vi "T3AWG Setup.vi"(4 "exact setup (True)":bool=TRUE, 5 "fs [Hz]":dbl=1000000000.0, 6 "N":i32, 7 "f [Hz]":dbl[](array[numeric]) format="%#_13g", 8 "error in (no error)":errorcluster, 9 "phi [deg]":dbl[](array[numeric]), 10 "A [-]":dbl[](array[numeric]), 11 "t3awg":T1 {"t3awg fs rules"."fs-step [Hz]" format="%#_6p"; "t3awg fs rules"."fs-max [Hz]" format="%#_6p"; "t3awg fs rules"."for f0 <" format="%#_6p"; "t3awg fs rules"."fs-min [Hz]" format="%#_6p"}) -> (0 "error out":errorcluster, 3 "t3awg out":T1 {"t3awg fs rules"."fs-step [Hz]" format="%#_6p"; "t3awg fs rules"."fs-max [Hz]" format="%#_6p"; "t3awg fs rules"."for f0 <" format="%#_6p"; "t3awg fs rules"."fs-min [Hz]" format="%#_6p"})   [LabVIEW 2020, in "Active Technologies AWG3000.lvlib"]
uses:
  Active Technologies AWG3000.lvlib
  T3AWG Session.ctl
  T3AWG Load Z.ctl
  fgen_ramdac_fs_rules.ctl
panel:
  in  "WaveGen Amplitude [Vpk] (3Vpk)":dbl=3.0 format="%#_13g"
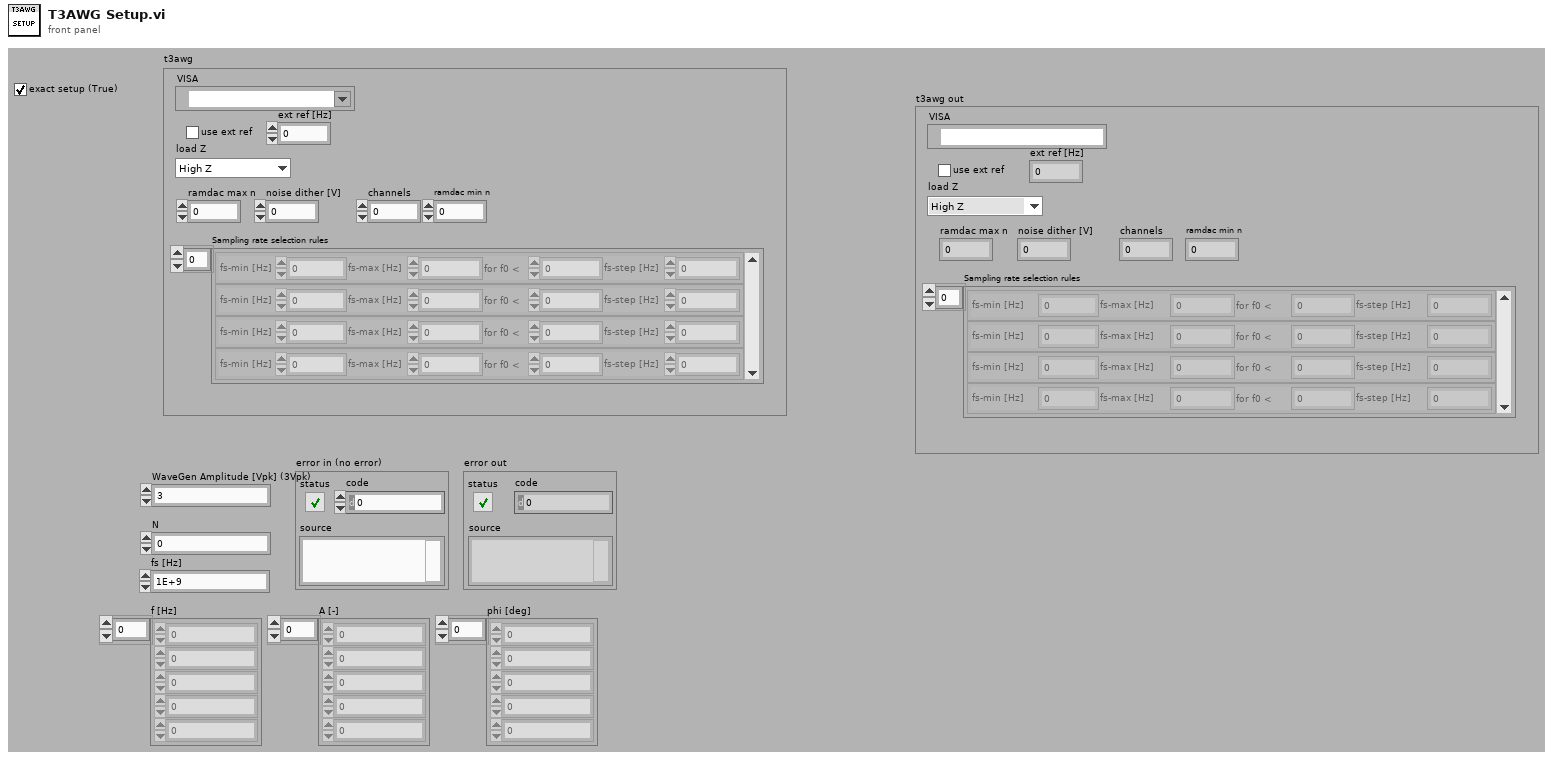
[diagram p1: front panel]
types:
  T1 = typedef "Active Technologies AWG3000.lvlib/T3AWG Session.ctl" = cluster{"VISA":refnum<visa-resource-name>, "use ext ref":bool, "ext ref [Hz]":dbl, "load Z":T2, "ramdac max n":i32, "noise dither [V]":dbl, "t3awg fs rules":T3[], "channels":i32, "ramdac min n":i32}
  T2 = typedef "Active Technologies AWG3000.lvlib/T3AWG Load Z.ctl" = enum16{"High Z", "50 Ohm"}
  T3 = typedef "Active Technologies AWG3000.lvlib/fgen_ramdac_fs_rules.ctl" = cluster{"fs-min [Hz]":dbl, "fs-max [Hz]":dbl, "for f0 < ":dbl, "fs-step [Hz]":dbl}
  T4 = cluster{"Entry Length":i32, "Repetition Count":i32, "Infinite Repetitions":bool, "Channels":cluster{"Analog Waveform":string, "Amplitude [V]":dbl, "Offset [V]":dbl}[], "Digital Waveform":string}
  T5 = cluster{"Analog Waveform":string, "Amplitude [V]":dbl, "Offset [V]":dbl}
  T6 = cluster{"Entry Length":i32, "Repetition Count":i32, "Infinite Repetitions":bool, "Channels":cluster{"Analog Waveform":string, "Amplitude [V]":dbl, "Offset [V]":dbl}[], "Digital Waveform":string}[]
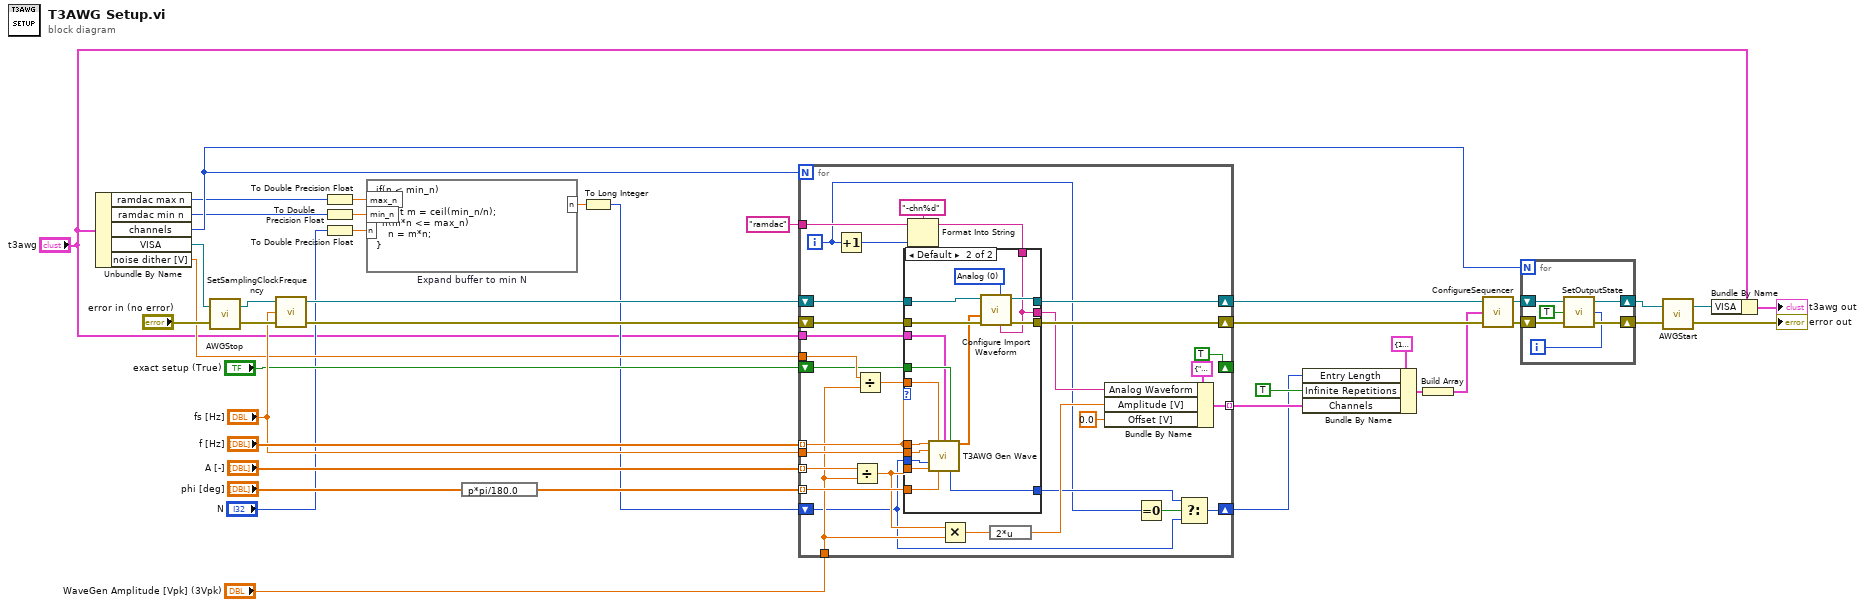
[diagram p0: block diagram]
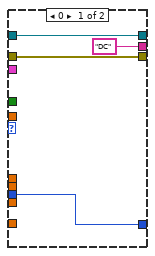
[diagram p2: hidden frame]
diagram:
  n1 = Unbundle By Name("t3awg") -> ("ramdac max n"=w8:i32, "ramdac min n"=w9:i32, "channels"=w17:i32, "VISA"=w38:refnum<visa-resource-name>, "noise dither [V]"=w12:dbl)
  n2 = call "AWGStop.vi"("error in (no error)"="error in (no error)", "VISA resource name"=w38) -> ("error out"=w37:errorcluster, "VISA resource name out"=w36:refnum<visa-resource-name>)
  n3 = call "SetSamplingClockFrequency.vi"("error in (no error)"=w37, "Sampling Clock (Hz)"="fs [Hz]", "VISA resource name"=w36) -> ("error out"=w25:errorcluster, "VISA resource name out"=w24:refnum<visa-resource-name>)  [unwired: 1 in]
  n4 = To Double Precision Float(number=w8) -> (double precision float=w7:dbl)
  n5 = To Double Precision Float(number=w9) -> (double precision float=w6:dbl)
  n6 = To Double Precision Float(number="N") -> (double precision float=w5:dbl)
  n7 = formula code="if(n < min_n)\n{\n  float m = ceil(min_n/n);\n  if(m*n <= max_n)\n    n = m*n;\n}" "Expand buffer to min N"("max_n"=w7, "min_n"=w6, "n"=w5) -> ("n"=w4:dbl)
  n8 = expression code="p*pi/180.0"("phi [deg]") -> (w26:dbl[])
  n9 = To Long Integer(number=w4) -> (32bit integer=w2:i32)
  n10 = for {
    N: w17 -> [_]
    tunnel: "f [Hz]" -> [w58] mode=indexing
    tunnel: "fs [Hz]" -> [w68]
    tunnel: "A [-]" -> [w55] mode=indexing
    shift-right: [w66] -> w21
    shift-left: w24 -> [w70]
    shift-right: [w67] -> w22
    shift-left: w25 -> [w69]
    tunnel: "ramdac" ("Set Waveform Name") -> [w65]
    tunnel: "WaveGen Amplitude [Vpk] (3Vpk)" -> [w49]
    tunnel: [w60] -> w29 mode=indexing
    tunnel: w26 -> [w59] mode=indexing
    tunnel: w12 -> [w51]
    shift-right: [w47] -> w10
    shift-left: w2 -> [w45]
    shift-right: [TRUE ("exact setup (True)")] -> _
    shift-left: "exact setup (True)" -> [w48]
    tunnel: "t3awg" -> [w41]
    i -> [w43]
    n11 = Increment(x=w43) -> (x+1=w63:i32)
    n12 = Divide(x=w55, y=w49) -> (x/y=w52:dbl)
    n13 = Divide(x=w51, y=w49) -> (x/y=w50:dbl)
    n14 = Format Into String(format string="-chn%d", initial string=w65, w63) -> (resulting string=w56:string)  [unwired: 1 in, 1 out]
    n15 = case shown="Default" w58 {
      tunnel: w70 -> [w73 w84]
      tunnel: w69 -> [w74 w85]
      tunnel: w58 -> [_ w90]
      tunnel: w68 -> [_ w89]
      tunnel: w52 -> [_ w88]
      tunnel: w45 -> [w71 w87]
      tunnel: [w74 w83] -> w67
      tunnel: [w73 w80] -> w66
      tunnel: ["DC" w78] -> w57
      tunnel: w59 -> [_ w86]
      tunnel: w56 -> [_ w78]
      tunnel: w50 -> [_ w79]
      tunnel: w48 -> [_ w77]
      tunnel: [w71 w76] -> w46
      tunnel: w41 -> [_ w75]
      frame 0 {
      }
      frame Default {
        w82 = u16 0 items=["Analog", "Digitals"] ("Specify the  Waveform Type")
        n16 = call "T3AWG Gen Wave.vi"("f [Hz]"=w90, "A-dither [-]"=w79, "t3awg"=w75, "exact setup (True)"=w77, "fs [Hz]"=w89, "N"=w87, "A [-]"=w88, "phi [rad]"=w86) -> ("wave"=w81:dbl[], "N out"=w76:i32)  [unwired: 3 in, 3 out]
        n17 = call "Configure Import Waveform.vi"("Set Waveform Name"=w78, "Specify the  Waveform Type"=w82, "error in (no error)"=w85, "wave in (range +/-1.0)"=w81, "VISA resource name"=w84) -> ("error out"=w83:errorcluster, "VISA resource name out"=w80:refnum<visa-resource-name>)  [unwired: 5 in]
      }
    }
    n18 = Multiply(x=w52, y=w49) -> (x*y=w53:dbl)
    n19 = expression code="2*u"(w53) -> (w54:dbl)
    n20 = Bundle By Name(cluster=T5 {"Analog Waveform"="", "Amplitude [V]"=0.0, "Offset [V]"=0.0} ("Cluster"), "Analog Waveform"=w57, "Amplitude [V]"=w54, "Offset [V]"=0.0) -> (w60:T5)
    n21 = Equal To 0?(x=w43) -> (x = 0?=w44:bool)
    n22 = Select(t=w46, s=w44, f=w45) -> (s? t:f=w47:i32)
  }
  n23 = Bundle By Name(cluster=T4 {"Entry Length"=16384, "Repetition Count"=1, "Infinite Repetitions"=FALSE, "Channels"=[{"Analog Waveform"="SINE", "Amplitude [V]"=0.0, "Offset [V]"=0.0}, {"Analog Waveform"="SINE", "Amplitude [V]"=0.0, "Offset [V]"=0.0}], "Digital Waveform"=""} ("Sequencer Item"), "Entry Length"=w10, "Infinite Repetitions"=TRUE, "Channels"=w29) -> (w31:T4)
  n24 = Build Array(w31) -> (w20:T6)
  n25 = call "ConfigureSequencer.vi"("error in (no error)"=w22, "Sequencer"=w20, "VISA resource name"=w21) -> ("error out"=w19:errorcluster, "VISA resource name out"=w18:refnum<visa-resource-name>)  [unwired: 1 in]
  n26 = for {
    N: w17 -> [_]
    shift-right: [w94] -> w16
    shift-left: w19 -> [w96]
    shift-right: [w91] -> w15
    shift-left: w18 -> [w95]
    i -> [w93]
    n27 = call "SetOutputState.vi"("Channel (0: Channel 1)"=w93, "error in (no error)"=w96, "Output State"=TRUE, "VISA resource name"=w95) -> ("error out"=w94:errorcluster, "VISA resource name out"=w91:refnum<visa-resource-name>)
  }
  n28 = call "AWGStart.vi"("error in (no error)"=w16, "VISA resource name"=w15) -> ("error out"=→"error out":errorcluster, "VISA resource name out"=w13:refnum<visa-resource-name>)
  n29 = Bundle By Name(cluster="t3awg", "VISA"=w13) -> (→"t3awg out":T1)
